vi "Unregister For Event.vi"(8 "Error In":errorcluster, 9 "Event Name":string, 10 "Registrant Address":refnum<class "Message Enqueuer.lvclass">, 11 "Event Source Actor In":refnum<class "Event Source Actor.lvclass">) -> (0 "Error Out":errorcluster, 3 "Event Source Actor Out":refnum<class "Event Source Actor.lvclass">)   [LabVIEW 2020, in "Event Source.lvlib" / "Event Source Actor.lvclass"]
doc: "This method unregisters a specific Actors Enqueuer from specific Event he is listening to, in this Event Source Actor."
uses:
  Event Source Actor.lvclass
  <vilib>/ActorFramework/Message Enqueuer/Message Enqueuer.lvclass
  Event Source Actor.lvclass/Event Source Actor.ctl
  c8cb1f89-adbf-4be7-8ea2-29bcf479b04f.vi
  Program Files/National Instruments/LabVIEW 2020/resource/AFDebug/AF Debug.lvlib
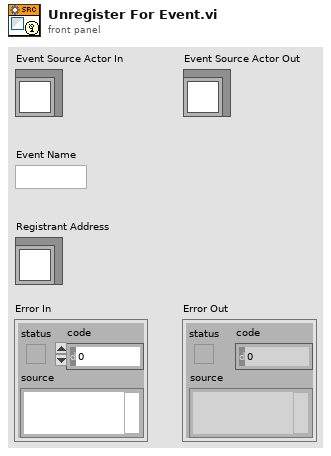
[diagram p1: front panel]
types:
  T1 = map{string, set{refnum<class "Message Enqueuer.lvclass">}}
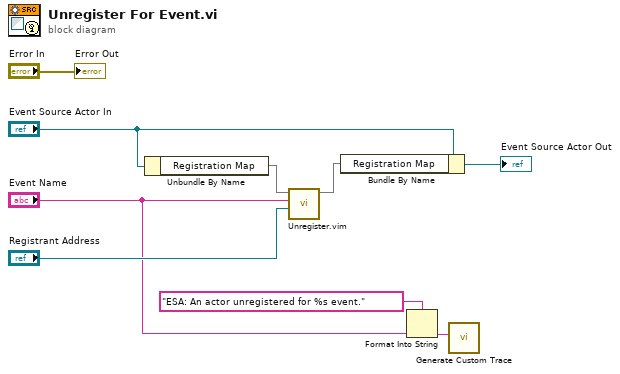
[diagram p0: block diagram]
diagram:
  n1 = Unbundle By Name("Event Source Actor In") -> ("Registration Map"=w9:T1)
  n2 = call "Unregister.vim"("set element"="Registrant Address", "key"="Event Name", "map in"=w9) -> ("map out"=w6:T1)  [unwired: 6 in, 2 out]
  n3 = Bundle By Name(cluster="Event Source Actor In", "Registration Map"=w6) -> (→"Event Source Actor Out":refnum<class "Event Source Actor.lvclass">)
  n4 = Format Into String(format string="ESA: An actor unregistered for %s event." ("Custom Action"), "Event Name") -> (resulting string=w2:string)  [unwired: 2 in, 1 out]
  n5 = call "Generate Custom Trace.vi"("Custom Action"=w2) -> ()  [unwired: 11 in]
  "Error Out" <- "Error In"
